vi "getNewestRow.vi"(10 "Rows":i32, 11 "Array":string[][](array[string])) -> (3 "Top Left Visible Cell":T1)   [LabVIEW 2015]
uses:
  <vilib>/Utility/miscctls.llb/LVRowAndColumnUnsignedTypeDef.ctl
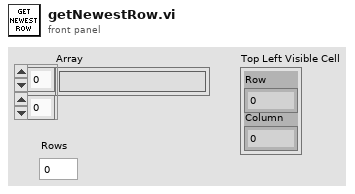
[diagram p1: front panel]
types:
  T1 = typedef "LVRowAndColumnUnsignedTypeDef.ctl" = cluster{"Row":u32, "Column":u32}
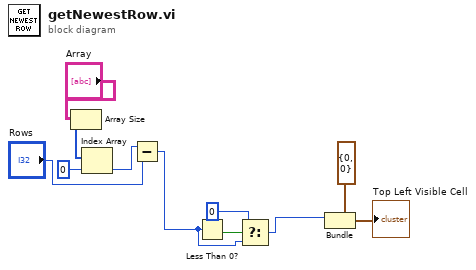
[diagram p0: block diagram]
diagram:
  n1 = Array Size(array="Array") -> (size(s)=w7:i32[])
  n2 = Index Array(array=w7, index=0) -> (element=w11:i32)
  n3 = Subtract(x=w11, y="Rows") -> (x-y=w3:i32)
  n4 = Less Than 0?(x=w3) -> (x < 0?=w4:bool)
  n5 = Select(t=0, s=w4, f=w3) -> (s? t:f=w1:i32)
  n6 = Bundle(cluster=T1 {"Row"=0, "Column"=0} ("Top Left Visible Cell"), "Row"=w1) -> (→"Top Left Visible Cell":T1)  [unwired: 1 in]
